vi "2DstrTableTodblArray.vi"(11 "strTable":string[][](table)) -> (3 "dbl2DArray":dbl[][](array[numeric]))   [LabVIEW 2014, in "Framework.lvlib"]
uses:
  Framework.lvlib
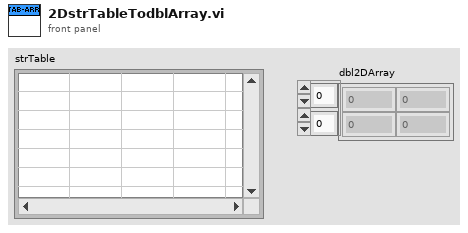
[diagram p1: front panel]
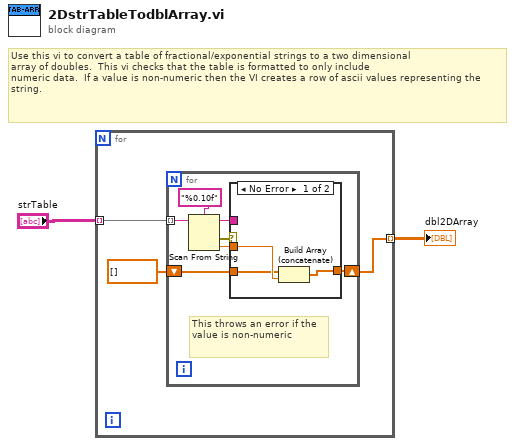
[diagram p0: block diagram]
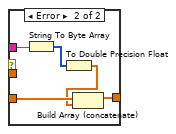
[diagram p2: hidden frame]
diagram:
  # "Use this vi to convert a table of fractional/exponential strings to a two dimensional\narray of doubles.  This vi checks that the table is formatted to only include\nnumeric data.  If a value is non-numeric then the VI creates a row of ascii values representing the string."
  n1 = for {
    tunnel: "strTable" -> [w5] mode=indexing
    tunnel: [w4] -> w2 mode=indexing
    n2 = for {
      tunnel: w5 -> [w12] mode=indexing
      shift-right: [w8] -> w4
      shift-left: dbl[] [] -> [w6]
      # "This throws an error if the value is non-numeric"
      n3 = Scan From String(format string="%0.10f", input string=w12) -> (remaining string=w7:string, error out=w10:errorcluster, output 1=w9:dbl)  [unwired: 3 in, 1 out]
      n4 = case shown="No Error" w10 {
        tunnel: w9 -> [w15 _]
        tunnel: [w13 w17] -> w8
        tunnel: w7 -> [_ w20]
        tunnel: w6 -> [w14 w18]
        frame No Error {
          n5 = Build Array (concatenate)(w14, w15) -> (w13:dbl[])
        }
        frame Error {
          n6 = String To Byte Array(string=w20) -> (unsigned byte array=w19:u8[])
          n7 = To Double Precision Float(number=w19) -> (double precision float=w16:dbl[])
          n8 = Build Array (concatenate)(w18, w16) -> (w17:dbl[])
        }
      }
    }
  }
  "dbl2DArray" <- w2
